vi "Get Histogram Style.vi"(8 "Error In":errorcluster, 10 "Plot Index":i32, 11 "Histogram Graph Refnum":refnum<vi>) -> (0 "Error Out":errorcluster, 2 "Updated Plot Info":T1={"Plot Index"=-1, "Plot Name"="", "# Plots"=0, "Plot Style"={"Plot Style"=enum."Histogram + Symbol", "Histogram Type"=enum."Right Bound", "Line Tickness"=enum."unchanged", "Line Style"=enum."unchanged", "Point Style"=enum."unchanged", "Line Color"=0, "Point Color"=0, "Anti-aliased"=FALSE, "Line Color Chooser"=enum."unchanged", "Point Color Chooser"=enum."unchanged", "Line Color List"="", "Point Color List"=""}})   [LabVIEW 2021, in "Histogram Window.lvlib"]
uses:
  Histogram Window.lvlib
  Histogram Updated Plot Info.ctl
  Graphs/Plot Style 3.ctl
  Graphs/Graphs.lvlib
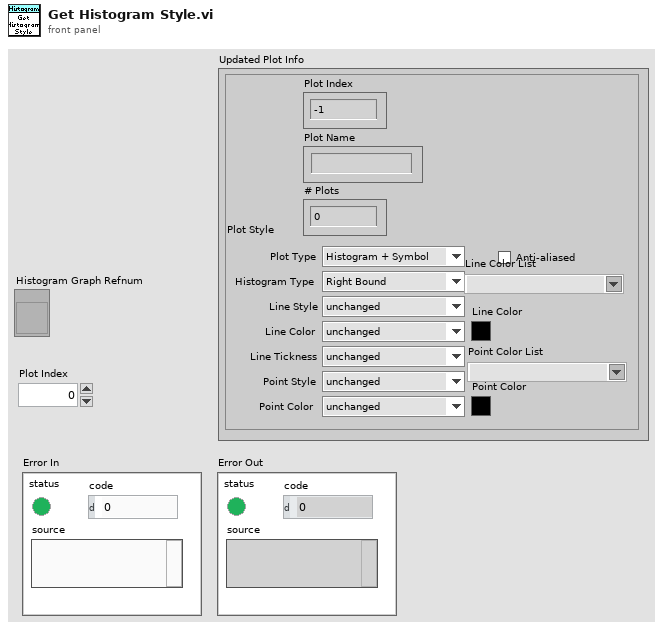
[diagram p1: front panel]
types:
  T1 = typedef "Histogram Window.lvlib/Histogram Updated Plot Info.ctl" = cluster{"Plot Index":i32, "Plot Name":string, "# Plots":i32, "Plot Style":T2}
  T2 = typedef "Graphs.lvlib/Plot Style 3.ctl" = cluster{"Plot Style":enum16{"unchanged", "Line", "Symbol", "Line + Symbol", "Histogram", "Histogram + Symbol"}, "Histogram Type":enum16{"unchanged", "Left Bound", "Center", "Right Bound"}, "Line Tickness":enum16{"unchanged", "Thin", "1 pixel", "2 pixel", "3 pixel", "4 pixel", "5 pixel"}, "Line Style":enum16{"unchanged", "Plain", "Long Dash", "Short Dash", "Long-Short Dash", "Long-Short-Short Dash"}, "Point Style":enum16{"unchanged", "None", "Empty Circle", "Filled Circle", "Thick Circle", "Dotted Circle", "Empty Square", "Filled Square", "Thick Square", "Dotted Square", "Small Filled Square", "Dot", "Cross", "Tiny Cross", "Large X", "Small x", "Diamond", "Small Empty Square"}, "Line Color":u32, "Point Color":u32, "Anti-aliased":bool, "Line Color Chooser":enum16{"unchanged", "Color Box", "Color List"}, "Point Color Chooser":enum16{"unchanged", "Color Box", "Color List"}, "Line Color List":string, "Point Color List":string}
  T3 = enum16{"unchanged", "Line", "Symbol", "Line + Symbol", "Histogram", "Histogram + Symbol"}
  T4 = enum16{"unchanged", "Left Bound", "Center", "Right Bound"}
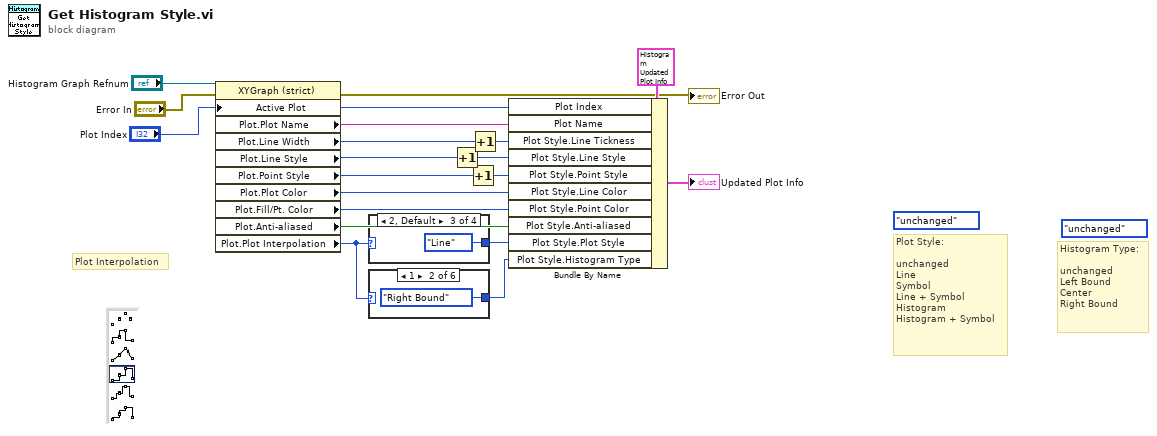
[diagram p0: block diagram]
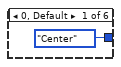
[diagram p2: hidden frame]
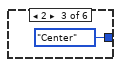
[diagram p3: hidden frame]
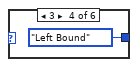
[diagram p4: hidden frame]
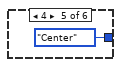
[diagram p5: hidden frame]
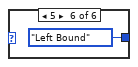
[diagram p6: hidden frame]
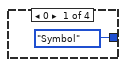
[diagram p7: hidden frame]
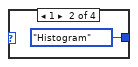
[diagram p8: hidden frame]
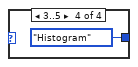
[diagram p9: hidden frame]
diagram:
  (unwired) T3."unchanged" ("Plot Style.Plot Style")
  (unwired) T4."unchanged" ("Plot Style.Histogram Type")
  # "Histogram Type:\n\nunchanged\nLeft Bound\nCenter\nRight Bound"
  # "Plot Style:\n\nunchanged\nLine\nSymbol\nLine + Symbol\nHistogram\nHistogram + Symbol"
  # "Plot Interpolation"
  n1 = property class="XYGraph (strict)"(reference="Histogram Graph Refnum", error in="Error In", "Active Plot"="Plot Index") -> (error out=→"Error Out":errorcluster, "Plot.Plot Name"=w16:string, "Plot.Line Width"=w15:u8, "Plot.Line Style"=w14:u8, "Plot.Point Style"=w11:u8, "Plot.Plot Color"=w9:u32, "Plot.Fill/Pt. Color"=w8:u32, "Plot.Anti-aliased"=w7:bool, "Plot.Plot Interpolation"=w2:u8)  [unwired: 1 out]
  n2 = case shown="2, Default" w2 {
    tunnel: [T3."Symbol" ("Plot Style.Plot Style") T3."Histogram" ("Plot Style.Plot Style") T3."Line" ("Plot Style.Plot Style") T3."Histogram" ("Plot Style.Plot Style")] -> w3
    frame 0 {
    }
    frame 1 {
    }
    frame 2, Default {
    }
    frame 3..5 {
    }
  }
  n3 = case shown="1" w2 {
    tunnel: [T4."Center" ("Plot Style.Histogram Type") T4."Right Bound" ("Plot Style.Histogram Type") T4."Center" ("Plot Style.Histogram Type") T4."Left Bound" ("Plot Style.Histogram Type") T4."Center" ("Plot Style.Histogram Type") T4."Left Bound" ("Plot Style.Histogram Type")] -> w1
    frame 0, Default {
    }
    frame 1 {
    }
    frame 2 {
    }
    frame 3 {
    }
    frame 4 {
    }
    frame 5 {
    }
  }
  n4 = Increment(x=w14) -> (x+1=w12:u8)
  n5 = Increment(x=w11) -> (x+1=w10:u8)
  n6 = Increment(x=w15) -> (x+1=w13:u8)
  n7 = Bundle By Name(cluster=T1 {"Plot Index"=-1, "Plot Name"="", "# Plots"=0, "Plot Style"={"Plot Style"=enum."Histogram + Symbol", "Histogram Type"=enum."Right Bound", "Line Tickness"=enum."unchanged", "Line Style"=enum."unchanged", "Point Style"=enum."unchanged", "Line Color"=0, "Point Color"=0, "Anti-aliased"=FALSE, "Line Color Chooser"=enum."unchanged", "Point Color Chooser"=enum."unchanged", "Line Color List"="", "Point Color List"=""}} ("Updated Plot Info"), "Plot Index"="Plot Index", "Plot Name"=w16, "Plot Style.Line Tickness"=w13, "Plot Style.Line Style"=w12, "Plot Style.Point Style"=w10, "Plot Style.Line Color"=w9, "Plot Style.Point Color"=w8, "Plot Style.Anti-aliased"=w7, "Plot Style.Plot Style"=w3, "Plot Style.Histogram Type"=w1) -> (→"Updated Plot Info":T1)
